vi "MultiChannelType_2D-Array-EXT.vi"(9 "error in":errorcluster, 11 "Array in":ext[][](array[numeric])) -> (1 "error out":errorcluster, 2 "MultiChannelType":cxt, 3 "Array out":ext[][](array[numeric]))   [LabVIEW 2020, in "OpenLvVision_OpenCv.lvlib"]
uses:
  OpenLvVision_OpenCv.lvlib
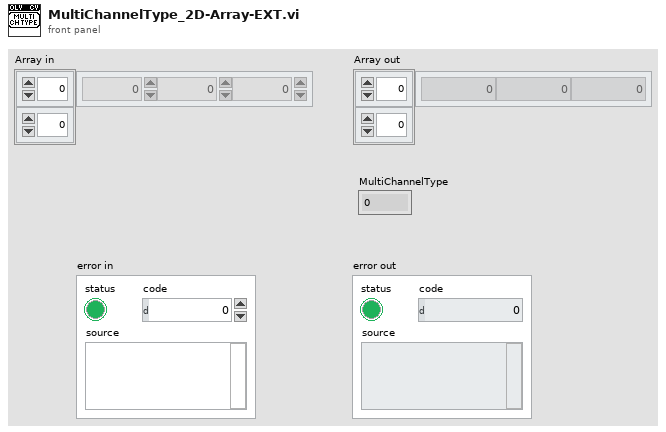
[diagram p1: front panel]
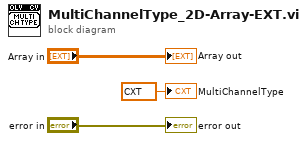
[diagram p0: block diagram]
diagram:
  "error out" <- "error in"
  "Array out" <- "Array in"
  "MultiChannelType" <- cxt 0.0+0.0i
